vi "CoordinateConvert_ArmToCartesian_Arrays.vi"(1 "ArmCoordinates":T2[](array[typedef])) -> (0 "XYPoints":T1[](array[typedef]))   [LabVIEW 2017]
uses:
  TypeDefs/ArmCoordinate.ctl
  General/PathPlanning/TypeDefs/Point2D.ctl
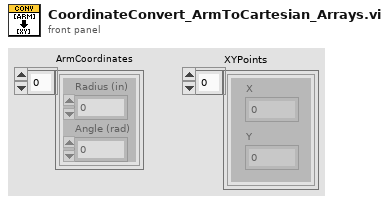
[diagram p1: front panel]
types:
  T1 = typedef "Point2D.ctl" = cluster{"X":dbl, "Y":dbl}
  T2 = typedef "ArmCoordinate.ctl" = cluster{"Radius (in)":dbl, "Angle (rad)":dbl}
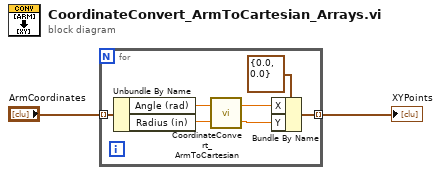
[diagram p0: block diagram]
diagram:
  n1 = for {
    tunnel: "ArmCoordinates" -> [w9] mode=indexing
    tunnel: [w3] -> w1 mode=indexing
    n2 = Unbundle By Name(w9) -> ("Angle (rad)"=w8:dbl, "Radius (in)"=w7:dbl)
    n3 = call "CoordinateConvert_ArmToCartesian.vi"("Radius (in)"=w7, "Angle (rad)"=w8) -> ("Y (in)"=w5:dbl, "X (in)"=w6:dbl)
    n4 = Bundle By Name(cluster=T1 {"X"=0.0, "Y"=0.0} ("2DPoint"), "X"=w6, "Y"=w5) -> (w3:T1)
  }
  "XYPoints" <- w1
